vi "Write.vi"(8 "error in (no error)":errorcluster, 10 "Text":string, 11 "Log in":refnum<class "Log.lvclass">) -> (0 "error out":errorcluster, 3 "Log out":refnum<class "Log.lvclass">)   [LabVIEW 2026, in "TALOS.lvlib" / "Classes.lvlib" / "Log.lvclass"]
uses:
  Log.lvclass
  Log.lvclass/Log.ctl
  Ancestor/Ancestor/Ancestor.lvclass/Ancestor.ctl
  FGV/Error Memory/Get Error Description.vi
  Support VIs/Get PC name.vi
  Ancestor/Ancestor/Read ID.vi
  Support VIs/Get Class Name.vi
  <vilib>/Utility/error.llb/Clear Errors.vi
  FGV/Error Memory/Error Memory Core.vi
  <vilib>/AdvancedString/Delimited String to 1D String Array.vi
  <vilib>/AdvancedString/Delimited String to 1D String Array (string).vi
  Support VIs/Circus Root Path.vi
  FGV/Error Memory/Error Crt Lvl checker.vi
  FGV/Error Memory/Error Memory Core.vi/40c8088d-b597-4017-91af-faa98e00292e.vi
  FGV/Error Memory/Error Memory Core.vi/d4a3ab98-063c-4e44-b43d-fbdcfe6c2be2.vi
  Support VIs/Global Memory.vi
  <vilib>/Utility/LVClass/Get LV Class Name.vi
  Support VIs/Is in Packed Library.vi
  Support VIs/TALOS Root path.vi
  Support VIs/Read CSV worksheet.vi
  Support VIs/Global Constants.vi
  <vilib>/Utility/error.llb/General Error Handler.vi
  Ancestor/Ancestor/Ancestor.lvclass
  <vilib>/Comparison/Equal/Equal Functor/Equal Functor.lvclass
  TALOS.lvlib
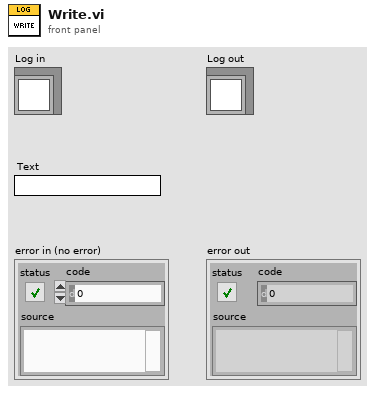
[diagram p1: front panel]
types:
  T1 = enum16{"open", "replace", "create", "open or create", "replace or create", "replace or create with confirmation"}
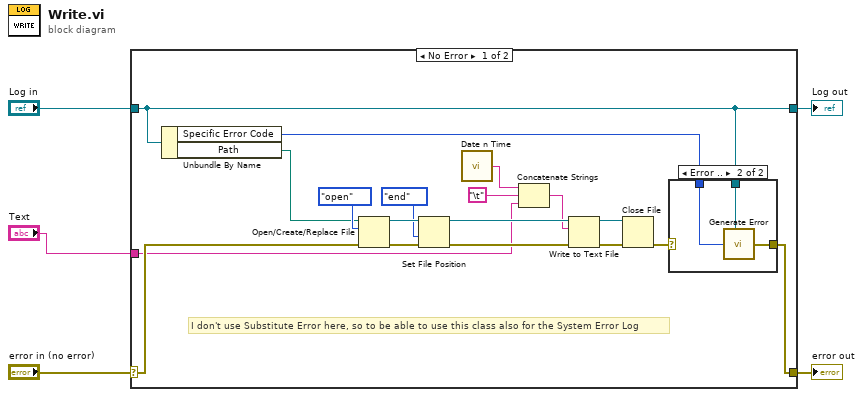
[diagram p0: block diagram]
diagram:
  n1 = case shown="No Error" "error in (no error)" {
    selector: "error in (no error)" -> [w19 w29]
    tunnel: [w11 w29] -> w2
    tunnel: [w9 w28] -> w4
    tunnel: "Log in" -> [w9 w28]
    tunnel: "Text" -> [w15 _]
    frame No Error {
      # "I don't use Substitute Error here, so to be able to use this class also for the System Error Log"
      n2 = Unbundle By Name(w9) -> ("Specific Error Code"=w10:i32, "Path"=w18:path)
      n3 = Open/Create/Replace File(file path (use dialog)=w18, error in=w19, operation (0:open)=T1."open") -> (refnum out=w23:refnum<file>, error out=w20:errorcluster)  [unwired: 3 in, 1 out]
      n4 = Set File Position(refnum=w23, from (0:start)=enum16{"start", "end", "current"}."end", error in=w20) -> (refnum out=w17:refnum<file>, error out=w16:errorcluster)  [unwired: 1 in]
      n5 = call "Date n Time.vi"() -> ("Date & Time"=w7:string)  [unwired: 5 in]
      n6 = Concatenate Strings(w7, "\t", w15) -> (w8:string)
      n7 = Write to Text File(file (use dialog)=w17, text=w8, error in=w16) -> (refnum out=w14:refnum<file>, error out=w13:errorcluster)  [unwired: 1 in, 1 out]
      n8 = Close File(refnum=w14, error in=w13) -> (error out=w12:errorcluster)  [unwired: 1 out]
      n9 = case shown="Error .." w12 {
        selector: w12 -> [w24 _]
        tunnel: [w24 w27] -> w11
        tunnel: w10 -> [_ w26]
        tunnel: w9 -> [_ w25]
        frame No Error {
        }
        frame Error {
          n10 = call "Generate Error.vi"("Class"=w25, "Error Code"=w26) -> ("error out"=w27:errorcluster)  [unwired: 5 in]
        }
      }
    }
    frame Error {
    }
  }
  "Log out" <- w4
  "error out" <- w2
